vi "Extract Profile Array.vi"(0 "Profile Data":u32[](array[numeric]), 5 "Profile Info":T1={"Profile Cnt"=1, "Envelope"=FALSE, " Profile Data Point"=0, " X Start"=0, " X Pitch"=0}, 7 "Profile Index (0)":u32, 9 "Profile Cnt (0: rest)":u32, 11 "error in (no error)":errorcluster) -> (4 "Profile A Array1":u32[][](array[numeric]), 6 "Profile B Array1":u32[][](array[numeric]), 8 "Profile A Array2":u32[][](array[numeric]), 10 "Profile B Array2":u32[][](array[numeric]), 15 "error out":errorcluster)   [LabVIEW 2014, in "Keyence LJ-V7000.lvlib"]
doc: "Only height data of profiles without a header and footer will be extracted to output in two-dimensional array from profile data acquired with VI such as <B>Read Profiles (for High-Speed Mode)</B> VI.\n\n<B>Note</B>:\nEmpty array will be output for corresponding output data if there is no profile data to extract."
uses:
  Keyence LJ-V7000.lvlib
  Clusters/Profile Info.ctl
panel:
  out "Extract Cnt for Debug":u32
  # "(c) 2012 KEYENCE CORPORATION.  ALL RIGHTS RESERVED."
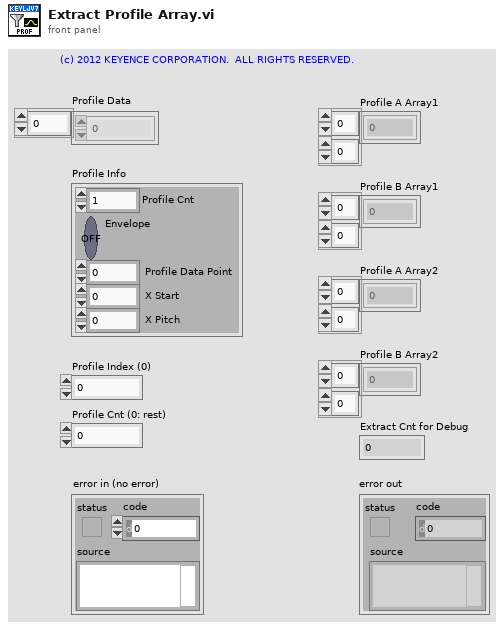
[diagram p1: front panel]
types:
  T1 = typedef "Keyence LJ-V7000.lvlib/Profile Info.ctl" = cluster{"Profile Cnt":u8, "Envelope":bool, " Profile Data Point":u16, " X Start":i32, " X Pitch":i32}
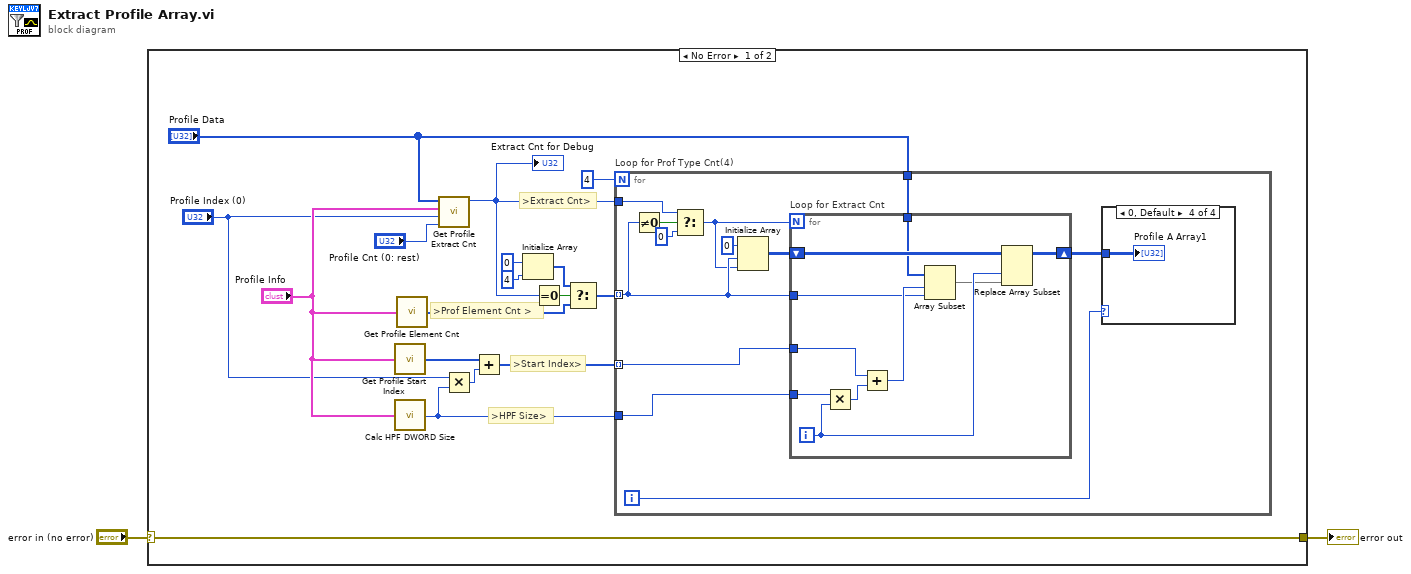
[diagram p0: block diagram]
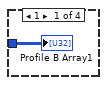
[diagram p2: hidden frame]
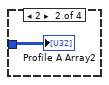
[diagram p3: hidden frame]
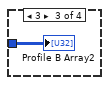
[diagram p4: hidden frame]
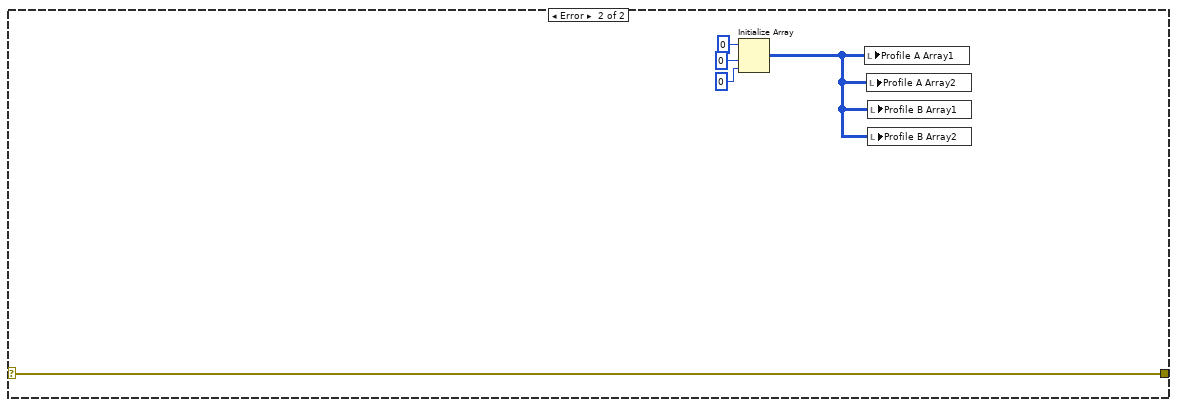
[diagram p5: hidden frame]
diagram:
  n1 = case shown="No Error" "error in (no error)" {
    selector: "error in (no error)" -> [w14 w50]
    tunnel: [w14 w50] -> w1
    frame No Error {
      # ">Start Index>"
      # ">HPF Size>"
      # ">Extract Cnt>"
      # ">Prof Element Cnt >"
      n2 = call "Get Profile Start Index.vi"("Profile Info"="Profile Info") -> ("Start Index[4]"=w15:u32[])  [unwired: 4 in]
      n3 = call "Calc HPF DWORD Size.vi"("Profile Info"="Profile Info") -> ("DWORD Size"=w17:u32)  [unwired: 4 in]
      n4 = call "Get Profile Element Cnt.vi"("Profile Info"="Profile Info") -> ("Element Cnt[4]"=w7:u16[])  [unwired: 4 in]
      n5 = call "Get Profile Extract Cnt.vi"("Profile Cnt (0: rest)"="Profile Cnt (0: rest)", "Profile Index (0)"="Profile Index (0)", "Profile Info"="Profile Info", "Profile Data"="Profile Data") -> ("Extract Cnt"=w8:u32)  [unwired: 7 in]
      "Extract Cnt for Debug" <- w8
      n6 = Multiply(x="Profile Index (0)", y=w17) -> (x*y=w16:u32)
      n7 = Add(x=w15, y=w16) -> (x+y=w18:u32[])
      n8 = Initialize Array(u16 0 ("要素"), 4 ("次元サイズ")) -> (w4:u16[])
      n9 = Equal To 0?(x=w8) -> (x = 0?=w9:bool)
      n10 = Select(t=w4, s=w9, f=w7) -> (s? t:f=w3:u16[])
      n11 = for "Loop for Prof Type Cnt(4)" {
        N: 4 -> [_]
        tunnel: w18 -> [w31] mode=indexing
        tunnel: w8 -> [w24]
        tunnel: w17 -> [w30]
        tunnel: "Profile Data" -> [w28]
        tunnel: w3 -> [w22] mode=indexing
        i -> [w26]
        n12 = Not Equal To 0?(x=w22) -> (x != 0?=w23:bool)
        n13 = Select(t=w24, s=w23, f=u32 0) -> (s? t:f=w20:u32)
        n14 = Initialize Array(u32 0, w22, w20) -> (w29:u32[][])
        n15 = for "Loop for Extract Cnt" {
          N: w20 -> [_]
          tunnel: w31 -> [w43]
          tunnel: w30 -> [w45]
          tunnel: w22 -> [w41]
          shift-right: [w39] -> w25
          shift-left: w29 -> [w38]
          tunnel: w28 -> [w37]
          i -> [w40]
          n16 = Multiply(x=w45, y=w40) -> (x*y=w44:u32)
          n17 = Add(x=w43, y=w44) -> (x+y=w42:u32)
          n18 = Array Subset ("部分配列")(array=w37, index=w42, length=w41) -> (w36:u32[])
          n19 = Replace Array Subset ("部分配列置換")(array=w38, new element=w36, index (col)=w40) -> (w39:u32[][])  [unwired: 1 in]
        }
        n20 = case shown="0, Default" w26 {
          tunnel: w25 -> [w32 w33 w34 w35]
          frame 1 {
            "Profile B Array1" <- w32
          }
          frame 2 {
            "Profile A Array2" <- w33
          }
          frame 3 {
            "Profile B Array2" <- w34
          }
          frame 0, Default {
            "Profile A Array1" <- w35
          }
        }
      }
    }
    frame Error {
      n21 = Initialize Array(u32 0 ("要素"), 0 ("次元サイズ"), 0 ("次元サイズ")) -> (w46:u32[][])
      n22 = local write "Profile A Array1"(w46) -> ()
      n23 = local write "Profile A Array2"(w46) -> ()
      n24 = local write "Profile B Array1"(w46) -> ()
      n25 = local write "Profile B Array2"(w46) -> ()
    }
  }
  "error out" <- w1
